vi "BonOMM-SAOMM.Test.vi"() -> ()   [LabVIEW 2011] (continued)
                                n1082 = Bundle("Angle Hor."=w4477, "DEC Tel"=w4476, "Epoch Tel"=w4468) -> (w4475:T29)  [unwired: 1 in]
                                n1083 = flat-sequence {
                                tunnel: w4483 -> [w4491]
                                tunnel: w4478 -> [w4490]
                                tunnel: w4475 -> [w4489]
                                tunnel: w4469 -> [w4488]
                                frame #0 {
                                n1084 = call "Hexapod-Console.vi"("CommCluster"=w4491, "ReferenceCluster"=w4490, "TelescopeCLuster"=w4489, "HexapodCluster"=w4488) -> ()  [unwired: 12 in]
                                }
                                frame #1 {
                                n1085 = local write "HexaSpam"(FALSE ("HexaSpam")) -> ()
                                }
                                }
                                n1086 = while {
                                stop <- w4494 continue-if-true
                                n1087 = Wait (ms)(milliseconds to wait=u32 500) -> ()  [unwired: 1 out]
                                n1088 = local read "HexaSpam"() -> (w4494:bool)
                                n1089 = property on="HexapodRefresh" class="Bool (strict)"("Val(Sgnl)"=TRUE ("Value (Signaling)")) -> ()  [unwired: 2 in, 2 out]
                                }
                                n1090 = Bundle("PrAMS actif"=w4482, "PrAMS-ACK"=w4479, "HexaCons actif"=w4480, "Hexapod-ACK"=w4481) -> (w4478:T30)  [unwired: 1 in]
                              }
                              frame Enabled {
                                n1091 = One Button Dialog(message="Fonction en développement ...\n\nUtilisez plutôt \"déplacement manuel\"") -> ()  [unwired: 1 in, 1 out]
                              }
                            }
                          }
                        }
                      }
                      frame "hex_Paramètres d'asservissement" {
                        # "Ici, on voudra probablement :\n  - Modifier la fréquence du filtre\n  - Modifier le nombre d'image prises en compte\n  - Modifier le coefficient d'aggressivité\n  - Modifier l'affichage de l'historique"
                        n1092 = One Button Dialog(message="Interaction usagé à définir ...") -> ()  [unwired: 1 in, 1 out]
                      }
                      frame "hex_Panneau de offset" {
                        n1093 = flat-sequence {
                          tunnel: [w4504] -> w4498
                          tunnel: w4498 -> [w4511]
                          frame #0 {
                            n1094 = local read "Mode"() -> (w4499:u16)
                            n1095 = case shown="Default" w4499 {
                              frame Default {
                              }
                              frame 0 {
                                n1096 = One Button Dialog(message="Il semble que le système ne soit pas en mode \"collimation\".\n\nPour que les valeurs de offsets demandés prennent effets, il\nest essentiel que le système soit en mode \"collimation\" ou \ntout autre mode utilisant l'hexapode.\n\nPour lancer le mode collimation, lancer d'abord l'exposition\nde la caméra de guidage puis sélectionné \"collimation\".\n\nL'application permettant de charger les offsets d'hexapode\nsera tout de même lancé, mais l'effet ne sera appliqué que\nlors du lancement d'un des modes utilisant l'hexapode.", button name ("OK")="J'ai lu et compris, merci.") -> ()  [unwired: 1 out]
                              }
                            }
                          }
                          frame #1 {
                            n1097 = local write "QueryingHexapod"(TRUE ("Value (Signaling)")) -> ()
                            n1098 = property on="HexapodRefresh" class="Bool (strict)"("Val(Sgnl)"=TRUE ("Value (Signaling)")) -> ()  [unwired: 2 in, 2 out]
                          }
                          frame #2 {
                            n1099 = while {
                              tunnel: [w4505] -> w4504
                              i -> [w4509]
                              stop <- w4508 stop-if-true
                              n1100 = local read "QueryingHexapod"() -> (w4505:bool)
                              n1101 = Not(x=w4505) -> (.not. x?=w4507:bool)
                              n1102 = Wait (ms)(milliseconds to wait=u32 100) -> ()  [unwired: 1 out]
                              n1103 = call "Max-iteration.vi"("i max"=50, "i act"=w4509, "Valeur entrante"=w4507) -> ("break ?"=w4508:bool)
                            }
                          }
                          frame #3 {
                            n1104 = case shown="False" w4511 {
                              frame False {
                                n1105 = control-ref of="Hexapod-ACK"() -> (w4514:refnum<vi>)
                                n1106 = local read "Hexapod VRN"() -> (w4515:refnum<visa-resource-name>)
                                n1107 = control-ref of="Offset X"() -> (w4518:refnum<vi>)
                                n1108 = control-ref of="Offset Y"() -> (w4519:refnum<vi>)
                                n1109 = control-ref of="Offset Z"() -> (w4520:refnum<vi>)
                                n1110 = control-ref of="Offset U"() -> (w4521:refnum<vi>)
                                n1111 = control-ref of="Offset V"() -> (w4522:refnum<vi>)
                                n1112 = local read "MessageType"() -> (w4512:cluster{string[], u32[]})
                                n1113 = control-ref of="HexaCons actif"() -> (w4513:refnum<vi>)
                                n1114 = Bundle("Offset X"=w4518, "Offset Y"=w4519, "Offset Z"=w4520, "Offset U"=w4521, "Offset V"=w4522) -> (w4517:T31)  [unwired: 1 in]
                                n1115 = call "TEST-SAOMM-OffsetGUI.vi"("Hexapod VRN"=w4515, "Active Refnum"=w4513, "PrAMS-ACK"=w4514, "output cluster"=w4517, "MessageType"=w4512) -> ("Error"=w4516:bool)  [unwired: 10 in]
                                n1116 = case shown="True" w4516 {
                                frame False {
                                }
                                frame True {
                                n1117 = One Button Dialog(message="Erreur lors de l'envoi\ndes valeurs de l'offset.") -> ()  [unwired: 1 in, 1 out]
                                }
                                }
                              }
                              frame True {
                                n1118 = One Button Dialog(message="Les valeurs de offsets n'ont pu être lu !?!\nVérifiez la connexion à \"hexapode-console\"") -> ()  [unwired: 1 in, 1 out]
                              }
                            }
                          }
                        }
                      }
                      frame "hex_Déplacement manuel" {
                        n1119 = flat-sequence {
                          tunnel: [w4528] -> w4525
                          tunnel: w4525 -> [w4535]
                          frame #0 {
                            n1120 = local write "QueryingHexapod"(TRUE ("Value (Signaling)")) -> ()
                            n1121 = property on="HexapodRefresh" class="Bool (strict)"("Val(Sgnl)"=TRUE ("Value (Signaling)")) -> ()  [unwired: 2 in, 2 out]
                          }
                          frame #1 {
                            n1122 = while {
                              tunnel: [w4529] -> w4528
                              i -> [w4533]
                              stop <- w4532 stop-if-true
                              n1123 = local read "QueryingHexapod"() -> (w4529:bool)
                              n1124 = Not(x=w4529) -> (.not. x?=w4531:bool)
                              n1125 = Wait (ms)(milliseconds to wait=u32 100) -> ()  [unwired: 1 out]
                              n1126 = call "Max-iteration.vi"("i max"=50, "i act"=w4533, "Valeur entrante"=w4531) -> ("break ?"=w4532:bool)
                            }
                          }
                          frame #2 {
                            n1127 = case shown="False" w4535 {
                              frame False {
                                n1128 = control-ref of="Hexapod-ACK"() -> (w4538:refnum<vi>)
                                n1129 = local read "Hexapod VRN"() -> (w4539:refnum<visa-resource-name>)
                                n1130 = control-ref of="HexX"() -> (w4542:refnum<vi>)
                                n1131 = control-ref of="HexY"() -> (w4543:refnum<vi>)
                                n1132 = control-ref of="HexZ"() -> (w4544:refnum<vi>)
                                n1133 = control-ref of="HexU"() -> (w4545:refnum<vi>)
                                n1134 = control-ref of="HexV"() -> (w4546:refnum<vi>)
                                n1135 = local read "MessageType"() -> (w4536:cluster{string[], u32[]})
                                n1136 = control-ref of="HexaCons actif"() -> (w4537:refnum<vi>)
                                n1137 = Bundle("HexX"=w4542, "HexY"=w4543, "HexZ"=w4544, "HexU"=w4545, "HexV"=w4546) -> (w4541:T28)  [unwired: 1 in]
                                n1138 = call "TEST-SAOMM-PositionGUI.vi"("Hexapod VRN"=w4539, "Active Refnum"=w4537, "PrAMS-ACK"=w4538, "output cluster"=w4541, "MessageType"=w4536) -> ("Error"=w4540:bool)  [unwired: 10 in]
                                n1139 = case shown="True" w4540 {
                                frame False {
                                }
                                frame True {
                                n1140 = One Button Dialog(message="Erreur lors de l'envoi\ndes valeurs de l'offset.") -> ()  [unwired: 1 in, 1 out]
                                }
                                }
                              }
                              frame True {
                                n1141 = One Button Dialog(message="Les valeurs de offsets n'ont pu être lu !?!\nVérifiez la connexion à \"hexapode-console\"") -> ()  [unwired: 1 in, 1 out]
                              }
                            }
                          }
                        }
                      }
                      frame "hex_Remise à zéro" {
                        n1142 = control-ref of="Hexapod-ACK"() -> (w4557:refnum<vi>)
                        n1143 = local read "Hexapod VRN"() -> (w4556:refnum<visa-resource-name>)
                        n1144 = local read "MessageType"() -> (w4553:cluster{string[], u32[]})
                        n1145 = control-ref of="HexaCons actif"() -> (w4558:refnum<vi>)
                        n1146 = local read "HexU"() -> (w4552:dbl)
                        n1147 = local read "HexV"() -> (w4551:dbl)
                        n1148 = local read "Signature"() -> (w4555:u32)
                        n1149 = local read "PrAMS Error"() -> (w4554:errorcluster)
                        n1150 = call "SAOMM-RaZ.vi"("PRAMMS-COMM IN"=w4556, "Active Refnum"=w4558, "PrAMS-ACK"=w4557, "Signature"=w4555, "Error IN"=w4554, "MessageType"=w4553, "Position U"=w4552, "Position V"=w4551) -> ("PRAMMS-COMM OUT"=w4550:refnum<visa-resource-name>, "Error OUT"=w4549:errorcluster)  [unwired: 6 in]
                        n1151 = local write "Hexapod VRN"(w4550) -> ()
                        n1152 = local write "PrAMS Error"(w4549) -> ()
                      }
                    }
                  }
                  frame "main_Caméra de référence" {
                    n1153 = case shown="\"cam_Modifier les paramètres\"" w4560 {
                      selector: w4560 -> [_ _ _ _ w4647 _]
                      tunnel: w4559 -> [_ _ _ _ _ _]
                      frame Default {
                      }
                      frame "cam_Enregistrer la prochaine image" {
                        n1154 = local write "SaveNextImage"(TRUE ("SaveNextImage")) -> ()
                      }
                      frame "cam_Modifier les paramètres" {
                        n1155 = flat-sequence {
                          tunnel: [w4601] -> w4568
                          tunnel: w4568 -> [w4614]
                          tunnel: [w4613] -> w4567
                          tunnel: [w4612] -> w4566
                          tunnel: [w4611] -> w4565
                          tunnel: [w4610] -> w4564
                          tunnel: [w4609] -> w4563
                          tunnel: [w4608] -> w4562
                          frame #0 {
                            n1156 = local write "QueryingPraMS"(TRUE ("Querying")) -> ()
                            n1157 = property on="FalconRefresh" class="Bool (strict)"("Val(Sgnl)"=TRUE ("Value (Signaling)")) -> ()  [unwired: 2 in, 2 out]
                          }
                          frame #1 {
                            n1158 = while {
                              tunnel: [w4603] -> w4601
                              i -> [w4607]
                              stop <- w4606 stop-if-true
                              n1159 = local read "QueryingPraMS"() -> (w4604:bool)
                              n1160 = Not(x=w4604) -> (.not. x?=w4603:bool)
                              n1161 = Wait Until Next ms Multiple(millisecond multiple=u32 50) -> ()  [unwired: 1 out]
                              n1162 = call "Max-iteration.vi"("i max"=100, "i act"=w4607, "Valeur entrante"=w4603) -> ("break ?"=w4606:bool)
                            }
                          }
                          frame #2 {
                            n1163 = case shown="True" w4614 {
                              tunnel: [FALSE ("Apply Changes") w4631] -> w4613
                              tunnel: [u16 0 ("Gain_OUT") w4630] -> w4612
                              tunnel: [u16 0 ("Binning_OUT") w4629] -> w4611
                              tunnel: [0.0 ("FPS_OUT") w4628] -> w4610
                              tunnel: [u16 0 ("Cooling_OUT") w4625] -> w4609
                              tunnel: [0 ("Binning_OUT") w4622] -> w4608
                              frame False {
                                n1164 = One Button Dialog(message="Problème de communication avec Prams") -> ()  [unwired: 1 in, 1 out]
                              }
                              frame True {
                                n1165 = local read "ImageFPS"() -> (w4632:dbl)
                                n1166 = property on="ROIsurface" class="Ring (strict)"() -> ("Strings []"=w4623:string[])  [unwired: 2 in, 2 out]
                                n1167 = local read "FPGA Value"() -> (w4626:u16)
                                n1168 = local read "ROIsurface"() -> (w4624:i32)
                                n1169 = local read "EMGain"() -> (w4627:u16)
                                n1170 = local read "Binning"() -> (w4633:u16)
                                n1171 = call "CameraSettings.vi"("Région d'intérêt"=w4624, "ROIStrings"=w4623, "Gain EM"=w4627, "Refroidissement"=w4626, "Binning"=w4633, "FPS"=w4632) -> ("Apply Changes"=w4631:bool, "Cooling_OUT"=w4625:u16, "Gain_OUT"=w4630:u16, "Binning_OUT"=w4629:u16, "ROISize_OUT"=w4622:i32, "FPS_OUT"=w4628:dbl)  [unwired: 4 in]
                              }
                            }
                          }
                        }
                        n1172 = case shown="True" w4567 {
                          tunnel: w4566 -> [_ w4582]
                          tunnel: w4565 -> [_ w4579]
                          tunnel: w4564 -> [_ w4575]
                          tunnel: w4563 -> [_ w4574]
                          tunnel: w4562 -> [_ w4570]
                          frame False {
                          }
                          frame True {
                            n1173 = flat-sequence {
                              tunnel: [w4588] -> w4583
                              tunnel: w4582 -> [w4588]
                              tunnel: [w4587] -> w4580
                              tunnel: w4579 -> [w4587]
                              tunnel: [w4586] -> w4576
                              tunnel: w4575 -> [w4586]
                              tunnel: w4574 -> [w4585]
                              tunnel: [w4584] -> w4571
                              tunnel: w4570 -> [w4584]
                              tunnel: w4583 -> [w4590]
                              tunnel: [w4592] -> w4581
                              tunnel: w4580 -> [w4592]
                              tunnel: [w4591] -> w4577
                              tunnel: w4576 -> [w4591]
                              tunnel: [w4589] -> w4572
                              tunnel: w4571 -> [w4589]
                              tunnel: w4581 -> [w4594]
                              tunnel: [w4595] -> w4578
                              tunnel: w4577 -> [w4595]
                              tunnel: [w4593] -> w4573
                              tunnel: w4572 -> [w4593]
                              tunnel: w4578 -> [w4597]
                              tunnel: w4573 -> [w4596]
                              tunnel: [w4596] -> w4569
                              tunnel: w4569 -> [w4598]
                              frame #0 {
                                n1174 = property on="FPGA Value" class="Ring (strict)"("Val(Sgnl)"=w4585) -> ()  [unwired: 2 in, 2 out]
                              }
                              frame #1 {
                                n1175 = property on="EMGain" class="DigNum (strict)"("Val(Sgnl)"=w4590) -> ()  [unwired: 2 in, 2 out]
                              }
                              frame #2 {
                                n1176 = property on="Binning" class="Ring (strict)"("Val(Sgnl)"=w4594) -> ()  [unwired: 2 in, 2 out]
                              }
                              frame #3 {
                                n1177 = property on="ImageFPS" class="DigNum (strict)"("Val(Sgnl)"=w4597) -> ()  [unwired: 2 in, 2 out]
                              }
                              frame #4 {
                                n1178 = property on="ROIsurface" class="Ring (strict)"("Val(Sgnl)"=w4598) -> ()  [unwired: 2 in, 2 out]
                              }
                            }
                          }
                        }
                      }
                      frame "cam_Modifier la région d'intérêt" {
                        n1179 = local read "ROIXOffset"() -> (w4644:u16)
                        n1180 = local read "ROIYOffset"() -> (w4643:u16)
                        n1181 = local read "ROIHeight"() -> (w4641:u16)
                        n1182 = local read "ROIWidth"() -> (w4642:u16)
                        n1183 = local read "ImgArray"() -> (w4639:u32[][])
                        n1184 = local read "ROISizes"() -> (w4640:u16[])
                        n1185 = property on="ROIsurface" class="Ring (strict)"() -> ("Strings []"=w4645:string[])  [unwired: 2 in, 2 out]
                        n1186 = call "ROISettings.vi"("ROISizes"=w4640, "SizeEnum"=w4645, "ImgArray"=w4639, "ROIHeight"=w4641, "ROIWidth"=w4642, "ROIYOffset"=w4643, "ROIXOffset"=w4644) -> ("ROIHeightOUT"=w4635:u16, "ROIWidthOUT"=w4636:u16, "ROIYOffsetOUT"=w4637:u16, "ROIXOffsetOUT"=w4638:u16, "SizesOUT"=w4634:i32)
                        n1187 = local write "ROIXOffset"(w4638) -> ()
                        n1188 = local write "ROIYOffset"(w4637) -> ()
                        n1189 = local write "ROIHeight"(w4635) -> ()
                        n1190 = local write "ROIWidth"(w4636) -> ()
                        n1191 = property on="ROIsurface" class="Ring (strict)"("Val(Sgnl)"=w4634) -> ()  [unwired: 2 in, 2 out]
                      }
                      frame "cam_Binning 1x1", "cam_Binning 2x2", "cam_Binning 4x4", "cam_Binning 5x5" {
                        n1192 = case shown="\"cam_Binning 1x1\"" w4647 {
                          tunnel: [u16 1 u16 1 u16 2 u16 4 u16 5] -> w4646
                          frame Default {
                          }
                          frame "cam_Binning 1x1" {
                          }
                          frame "cam_Binning 2x2" {
                          }
                          frame "cam_Binning 4x4" {
                          }
                          frame "cam_Binning 5x5" {
                          }
                        }
                        n1193 = property on="Binning" class="Ring (strict)"("Val(Sgnl)"=w4646) -> ()  [unwired: 2 in, 2 out]
                      }
                      frame "cam_Reconnexion" {
                        n1194 = One Button Dialog(message="Devrait reconnecter Prams ...") -> ()  [unwired: 1 in, 1 out]
                      }
                    }
                  }
                  frame "main_Tables de guidage" {
                    n1195 = case shown="\"tab_Commandes XYZ\"" w4654 {
                      frame Default {
                      }
                      frame "tab_Modifier les vitesses des tables" {
                        # "GUI pour modifier la vitesse des tales ..."
                        n1196 = local read "vitesse lente"() -> (w4660:dbl)
                        n1197 = local read "accelleration"() -> (w4659:dbl)
                        n1198 = local read "vitesse focus"() -> (w4656:dbl)
                        n1199 = local read "vitesse rapide"() -> (w4662:dbl)
                        n1200 = call "Set_table_speed.vi"("Z IN"=w4656, "Accel IN"=w4659, "Fast IN"=w4662, "slow IN"=w4660) -> ("Z OUT"=w4655:dbl, "Accel OUT"=w4657:dbl, "Fast OUT"=w4661:dbl, "slow OUT"=w4658:dbl)  [unwired: 4 in]
                        n1201 = local write "vitesse rapide"(w4661) -> ()
                        n1202 = local write "accelleration"(w4657) -> ()
                        n1203 = local write "vitesse focus"(w4655) -> ()
                        n1204 = local write "vitesse lente"(w4658) -> ()
                      }
                      frame "tab_Positions prédéfinies" {
                        n1205 = local read "Rangement X"() -> (w4672:dbl)
                        n1206 = local read "Rangement Y"() -> (w4673:dbl)
                        n1207 = local read "Rangement Z"() -> (w4671:dbl)
                        n1208 = local read "Calibration X"() -> (w4682:dbl)
                        n1209 = local read "Calibration Y"() -> (w4681:dbl)
                        n1210 = local read "Reference X"() -> (w4679:dbl)
                        n1211 = local read "Reference Y"() -> (w4678:dbl)
                        n1212 = local read "CentreTel X"() -> (w4676:dbl)
                        n1213 = local read "CentreTel Y"() -> (w4675:dbl)
                        n1214 = local read "Position X"() -> (w4670:dbl)
                        n1215 = local read "Position Y"() -> (w4669:dbl)
                        n1216 = Bundle("CentreTel X"=w4676, "CentreTel Y"=w4675) -> (w4674:cluster{"CentreTel X":dbl, "CentreTel Y":dbl})  [unwired: 1 in]
                        n1217 = Bundle("Reference X"=w4679, "Reference Y"=w4678) -> (w4677:cluster{"Reference X":dbl, "Reference Y":dbl})  [unwired: 1 in]
                        n1218 = Bundle("Calibration X"=w4682, "Calibration Y"=w4681) -> (w4680:T32)  [unwired: 1 in]
                        n1219 = Bundle("Rangement X"=w4672, "Rangement Y"=w4673, "Rangement Z"=w4671) -> (w4666:T33)  [unwired: 1 in]
                        n1220 = call "Set_predefined_table_positions.vi"("Calibration IN"=w4680, "Position Y"=w4669, "Position X"=w4670, "Reference IN"=w4677, "Centre IN"=w4674, "Park IN"=w4666) -> ("Calibration OUT"=w4667:T34, "Reference OUT"=w4663:cluster{"Reference Y":dbl, "Reference X":dbl}, "Centre OUT"=w4664:cluster{"Centre Y":dbl, "Centre X":dbl}, "Accept?"=w4668:bool, "Park OUT"=w4665:T35)  [unwired: 5 in]
                        n1221 = case shown="True" w4668 {
                          tunnel: w4667 -> [_ w4695]
                          tunnel: w4665 -> [_ w4692]
                          tunnel: w4664 -> [_ w4688]
                          tunnel: w4663 -> [_ w4685]
                          frame False {
                          }
                          frame True {
                            n1222 = Unbundle(w4695) -> ("Calibration Y"=w4694:dbl, "Calibration X"=w4693:dbl)
                            n1223 = Unbundle(w4688) -> ("Centre Y"=w4687:dbl, "Centre X"=w4686:dbl)
                            n1224 = Unbundle(w4685) -> ("Reference Y"=w4684:dbl, "Reference X"=w4683:dbl)
                            n1225 = Unbundle(w4692) -> ("Range Y"=w4691:dbl, "Range X"=w4690:dbl, "Range Z"=w4689:dbl)
                            n1226 = local write "Rangement X"(w4691) -> ()
                            n1227 = local write "Rangement Y"(w4690) -> ()
                            n1228 = local write "Rangement Z"(w4689) -> ()
                            n1229 = local write "Calibration X"(w4694) -> ()
                            n1230 = local write "Calibration Y"(w4693) -> ()
                            n1231 = local write "Reference X"(w4684) -> ()
                            n1232 = local write "Reference Y"(w4683) -> ()
                            n1233 = local write "CentreTel X"(w4687) -> ()
                            n1234 = local write "CentreTel Y"(w4686) -> ()
                          }
                        }
                      }
                      frame "tab_Commandes XYZ" {
                        n1235 = local read "MovingZ"() -> (w4698:bool)
                        n1236 = local read "MovingXY"() -> (w4697:bool)
                        n1237 = Or(x=w4698, y=w4697) -> (x .or. y?=w4696:bool)
                        n1238 = case shown="False" w4696 {
                          frame False {
                            n1239 = control-ref of="Table VRN"() -> (w4702:refnum<vi>)
                            n1240 = control-ref of="Table Error"() -> (w4701:refnum<vi>)
                            n1241 = control-ref of="Table actif"() -> (w4700:refnum<vi>)
                            n1242 = control-ref of="Cible X"() -> (w4705:refnum<vi>)
                            n1243 = control-ref of="Cible Y"() -> (w4706:refnum<vi>)
                            n1244 = control-ref of="Cible Z"() -> (w4704:refnum<vi>)
                            n1245 = local read "Position X"() -> (w4709:dbl)
                            n1246 = local read "Position Y"() -> (w4708:dbl)
                            n1247 = local read "Position Z"() -> (w4707:dbl)
                            n1248 = Bundle("Cible X"=w4705, "Cible Y"=w4706, "Cible Z"=w4704) -> (w4703:T36)  [unwired: 1 in]
                            n1249 = Bundle("Table VRN"=w4702, "Table Error"=w4701, "Table actif"=w4700) -> (w4699:T37)  [unwired: 1 in]
                            n1250 = call "CommandesXYZ.vi"("Structure-Communications"=w4699, "Structure-Cibles"=w4703, "Position X"=w4709, "Position Y"=w4708, "Position Z"=w4707) -> ()  [unwired: 11 in]
                          }
                          frame True {
                            n1251 = One Button Dialog(message="Les tables de translation semblent déjà être\nen mouvement, assurez-vous qu'elles sont arrêtées\navant de lancer le mode \"XYZ\".") -> ()  [unwired: 1 in, 1 out]
                          }
                        }
                      }
                      frame "tab_Modifier les paramètres" {
                        # "ClickJOG est en minute d'arc ..."
                        n1252 = local read "ClickJOG"() -> (w4714:dbl)
                        n1253 = expression code="x*60.0"(w4714) -> (w4713:dbl)
                        n1254 = call "Set-Jog-Params.vi"("clic IN"=w4713) -> ("clic OUT"=w4712:dbl)  [unwired: 14 in]
                        n1255 = expression code="x/60.0"(w4712) -> (w4711:dbl)
                        n1256 = local write "ClickJOG"(w4711) -> ()
                      }
                      frame "Reconnexion" {
                      }
                    }
                  }
                  frame "main_Roue à filtres" {
                    n1257 = case shown="\"raf_Reconnexion\"" w4715 {
                      selector: w4715 -> [w4721 _ _]
                      frame Default {
                        w4719 = "@@"
                        # "hmm, à compléter ...\n\n  - Cocher le filtre en place\n  - Commencer par rafraichir\n  - Si déconnecté, ne pas permettre un déplacement de la roue ..."
                        n1258 = Search/Split String(string=w4721, search string/char (-)=w4719) -> (match + rest of string=w4720:string)  [unwired: 1 in, 2 out]
                        n1259 = String Length(string=w4719) -> (length=w4718:i32)
                        n1260 = String Subset(string=w4720, offset (0)=w4718) -> (substring=w4717:string)  [unwired: 1 in]
                        n1261 = Decimal String To Number(string=w4717) -> (number=w4716:i32)  [unwired: 2 in, 1 out]
                        n1262 = Greater Or Equal To 0?(x=w4716) -> (x >= 0?=w4722:bool)
                        n1263 = case shown="True" w4722 {
                          tunnel: w4716 -> [_ w4734]
                          frame False {
                          }
                          frame True {
                            n1264 = Replace Array Subset(array=bool[] [FALSE, FALSE, FALSE, FALSE, FALSE, FALSE], new element=TRUE ("new element/subarray"), index=w4734) -> (w4728:bool[])
                            n1265 = property on="ChoixFiltre" class="Clust (strict)"() -> ("Value"=w4731:T12)  [unwired: 2 in, 2 out]
                            n1266 = Index Array(array=w4728) -> (element #1=w4729:bool, element #2=w4727:bool, element #3=w4726:bool, element #4=w4725:bool, element #5=w4724:bool, element #6=w4723:bool)  [unwired: 6 in]
                            n1267 = Bundle(cluster=w4731, "filtre #1"=w4729, "filtre #2"=w4727, "filtre #3"=w4726, "filtre #4"=w4725, "filtre #5"=w4724, "filtre #6"=w4723) -> (w4730:T12)
                            n1268 = property on="ChoixFiltre" class="Clust (strict)"("Val(Sgnl)"=w4730) -> ()  [unwired: 2 in, 2 out]
                          }
                        }
                      }
                      frame "raf_Modifier la liste des filtres" {
                        n1269 = flat-sequence {
                          frame #0 {
                            n1270 = local write "HautDroit"(T11."Périphérique" ("HautDroit")) -> ()
                          }
                          frame #1 {
                            n1271 = property on="change_filtre_liste" class="Bool (strict)"("Val(Sgnl)"=TRUE) -> ()  [unwired: 2 in, 2 out]
                          }
                        }
                      }
                      frame "raf_Reconnexion" {
                        n1272 = flat-sequence {
                          frame #0 {
                            w4738 = u16 0 items=["Roue à Filtres (BonOMM)", "Roue à Filtres (PANO-II)", "Foyer ST-133", "Lampes d'étalonnage", "Options des périphériques"] ("Périphérique")
                            n1273 = local write "HautDroit"(T11."Périphérique" ("HautDroit")) -> ()
                            n1274 = local write "Périphérique"(w4738) -> ()
                          }
                          frame #1 {
                            n1275 = property on="reconnect" class="Bool (strict)"("Val(Sgnl)"=TRUE ("Value (Signaling)")) -> ()  [unwired: 2 in, 2 out]
                          }
                        }
                      }
                    }
                  }
                }
              }
              event Key Down {
                n1276 = event-data() -> ("Char"=w4740:i16, "ScanCode"=w4741:i16)  [unwired: 1 in, 7 out]
                n1277 = case shown="0" w4740 {
                  tunnel: w4741 -> [_ w4742 _ _ _ _ _ _]
                  frame Default {
                    # "Do nothing ..."
                  }
                  frame 0 {
                    n1278 = case shown="72, 75, 77, 80" w4742 {
                      selector: w4742 -> [_ w4744]
                      frame Default {
                      }
                      frame 72, 75, 77, 80 {
                        # "Les 4 flèches ..."
                        # "Passer dans une astrométrie ?"
                        n1279 = local read "Servo"() -> (w4743:bool)
                        n1280 = case shown="False" w4743 {
                          tunnel: w4744 -> [w4758 _]
                          frame False {
                            # "Va marcher seulement 99.9% du temps, les SETs doivent être directement\nici si on veut éviter que ProcessedFalconImage ne puisse venir modifier\nles paramètres avant l'envoi."
                            n1281 = property on="ImgArray" class="IntGraph (strict)"("Active Cursor"=u32 0) -> (error out=w4755:errorcluster)  [unwired: 2 in, 1 out]
                            n1282 = property on="ImgArray" class="IntGraph (strict)"(error in=w4755) -> ("Cursor.Cursor X"=w4757:dbl, "Cursor.Cursor Y"=w4756:dbl)  [unwired: 1 in, 2 out]
                            n1283 = case shown="Default" w4758 {
                              tunnel: w4757 -> [w4763 w4764 w4768 w4772 w4775]
                              tunnel: w4756 -> [w4762 w4766 w4769 w4771 w4773]
                              tunnel: [w4763 w4764 w4767 w4772 w4774] -> w4753
                              tunnel: [w4762 w4765 w4769 w4770 w4773] -> w4752
                              frame Default {
                              }
                              frame 72 {
                                # "\"Up\""
                                n1284 = Increment(x=w4766) -> (x+1=w4765:dbl)
                              }
                              frame 77 {
                                # "\"Right\""
                                n1285 = Increment(x=w4768) -> (x+1=w4767:dbl)
                              }
                              frame 80 {
                                # "\"Down\""
                                n1286 = Decrement(x=w4771) -> (x-1=w4770:dbl)
                              }
                              frame 75 {
                                # "\"Left\""
                                n1287 = Decrement(x=w4775) -> (x-1=w4774:dbl)
                              }
                            }
                            n1288 = local read "ROIWidth"() -> (w4751:u16)
                            n1289 = local read "ROIHeight"() -> (w4750:u16)
                            n1290 = control-ref of="ImgArray"() -> (w4745:refnum<vi>)
                            n1291 = call "SAOMM-Cursor2ROI.vi"("ImgRef"=w4745, "CursorX"=w4753, "CursorY"=w4752, "ROIWidth"=w4751, "ROIHeight"=w4750) -> ("XÉtoile"=w4746:dbl, "YÉtoile"=w4747:dbl, "ROIXOffset"=w4749:u16, "ROIYOffset"=w4748:u16)  [unwired: 7 in]
                            n1292 = local write "XReference"(w4746) -> ()
                            n1293 = local write "YReference"(w4747) -> ()
                            n1294 = flat-sequence {
                              tunnel: w4749 -> [w4760]
                              tunnel: w4748 -> [w4759]
                              frame #0 {
                                n1295 = local write "ROIXOffset"(w4760) -> ()
                                n1296 = local write "ROIYOffset"(w4759) -> ()
                              }
                              frame #1 {
                                n1297 = property on="UpdateROI" class="Bool (strict)"("Val(Sgnl)"=TRUE ("Value (Signaling)")) -> ()  [unwired: 2 in, 2 out]
                              }
                            }
                          }
                          frame True {
                            n1298 = One Button Dialog(message="Vous ne pouvez pas modifier la ROI pendant l'asservissement") -> ()  [unwired: 1 in, 1 out]
                          }
                        }
                      }
                    }
                  }
                  frame 9 {
                    # "tab"
                    n1299 = property on="Offset OK" class="Bool (strict)"() -> ("Key Focus"=w4777:bool)  [unwired: 2 in, 2 out]
                    n1300 = property on="N.O. A.D." class="Str"() -> ("Key Focus"=w4781:bool)  [unwired: 2 in, 2 out]
                    n1301 = property on="N.O. Déc." class="Str"() -> ("Key Focus"=w4782:bool)  [unwired: 2 in, 2 out]
                    n1302 = property on="NO epoch" class="DigNum (strict)"() -> ("Key Focus"=w4783:bool)  [unwired: 2 in, 2 out]
                    n1303 = property on="ModCoor" class="Bool (strict)"() -> ("Key Focus"=w4784:bool)  [unwired: 2 in, 2 out]
                    n1304 = property on="Offset RA" class="DigNum (strict)"() -> ("Key Focus"=w4779:bool)  [unwired: 2 in, 2 out]
                    n1305 = property on="Offset DEC" class="DigNum (strict)"() -> ("Key Focus"=w4778:bool)  [unwired: 2 in, 2 out]
                    n1306 = Compound Arithmetic op=OR(w4781, w4782, w4783, w4784, w4779, w4778, w4777) -> (w4780:bool)
                    n1307 = case shown="False" w4780 {
                      frame False {
                        n1308 = flat-sequence {
                          frame #0 {
                            n1309 = property on="N.O. A.D." class="Str"("Key Focus"=TRUE) -> ()  [unwired: 2 in, 2 out]
                          }
                          frame #1 {
                            n1310 = property on="NO RA clic-sim" class="Bool (strict)"("Val(Sgnl)"=TRUE ("Value (Signaling)")) -> ()  [unwired: 2 in, 2 out]
                          }
                        }
                      }
                      frame True {
                      }
                    }
                  }
                  frame 32 {
                    # "Space bar"
                    n1311 = property on="Obslib" class="Tbl (strict)"() -> ("Key Focus"=w4787:bool)  [unwired: 2 in, 2 out]
                    n1312 = case shown="False" w4787 {
                      frame False {
                        n1313 = property on="Offset RA" class="DigNum (strict)"("Key Focus"=TRUE) -> ()  [unwired: 2 in, 2 out]
                      }
                      frame True {
                      }
                    }
                  }
                  frame 101 {
                    # "'e' pour Est"
                    n1314 = local read "Offset RA"() -> (w4790:dbl)
                    n1315 = Absolute Value(x=w4790) -> (abs(x)=w4789:dbl)
                    n1316 = property on="Offset RA" class="DigNum (strict)"("Val(Sgnl)"=w4789) -> ()  [unwired: 2 in, 2 out]
                  }
                  frame 110 {
                    # "'n' pour Nord"
                    n1317 = local read "Offset DEC"() -> (w4792:dbl)
                    n1318 = Absolute Value(x=w4792) -> (abs(x)=w4791:dbl)
                    n1319 = property on="Offset DEC" class="DigNum (strict)"("Val(Sgnl)"=w4791) -> ()  [unwired: 2 in, 2 out]
                  }
                  frame 111, 119 {
                    # "'o' ou 'w' pour Ouest"
                    n1320 = local read "Offset RA"() -> (w4795:dbl)
                    n1321 = Absolute Value(x=w4795) -> (abs(x)=w4794:dbl)
                    n1322 = Negate(x=w4794) -> (-x=w4793:dbl)
                    n1323 = property on="Offset RA" class="DigNum (strict)"("Val(Sgnl)"=w4793) -> ()  [unwired: 2 in, 2 out]
                  }
                  frame 115 {
                    # "'s' pour Sud"
                    n1324 = local read "Offset DEC"() -> (w4798:dbl)
                    n1325 = Absolute Value(x=w4798) -> (abs(x)=w4797:dbl)
                    n1326 = Negate(x=w4797) -> (-x=w4796:dbl)
                    n1327 = property on="Offset DEC" class="DigNum (strict)"("Val(Sgnl)"=w4796) -> ()  [unwired: 2 in, 2 out]
                  }
                }
              }
              event Mouse Move {
                n1328 = event-data() -> ()  [unwired: 1 in, 4 out]
                n1329 = disable-structure shown="Enabled" {
                  frame Disabled {
                    n1330 = while {
                      stop <- w4802 continue-if-true
                      w4803 = -1 ("x")
                      n1331 = property on="Picture" class="Pict"() -> ("Mouse"=w4806:T38)  [unwired: 2 in, 2 out]
                      n1332 = Unbundle By Name(w4806) -> ("Mouse Position.X"=w4801:i32, "Mouse Position.Y"=w4800:i32, "Mouse Modifiers.Button Down"=w4799:bool)
                      n1333 = case shown="True" w4799 {
                        frame False {
                        }
                        frame True {
                          n1334 = control-ref of="ImgArray"() -> (w4807:refnum<vi>)
                          n1335 = local write "Naxis1"(i16 640 ("Nx")) -> ()
                          n1336 = local write "Naxis2"(i16 480 ("Ny")) -> ()
                          n1337 = local write item#-1(i16 0 ("Xs")) -> ()
                          n1338 = local write item#-1(i16 0 ("Ys")) -> ()
                          n1339 = stacked-sequence {
                            seq-local: [w4813 _] -> [_ w4873]
                            seq-local: [w4812 _] -> [_ w4872]
                            tunnel: w4807 -> [w4814 _]
                            frame #0 {
                              n1340 = while {
                                tunnel: w4814 -> [w4817]
                                tunnel: [w4816] -> w4813
                                tunnel: [w4815] -> w4812
                                i -> [w4819]
                                stop <- w4818 continue-if-true
                                n1341 = property on="Picture" class="Pict"() -> ("Mouse"=w4821:T38)  [unwired: 2 in, 2 out]
                                n1342 = Equal To 0?(x=w4819) -> (x = 0?=w4820:bool)
                                n1343 = Unbundle By Name(w4821) -> ("Mouse Position.X"=w4816:i32, "Mouse Position.Y"=w4815:i32, "Mouse Modifiers.Button Down"=w4818:bool)
                                n1344 = case shown="False" w4820 {
                                tunnel: w4816 -> [w4823 w4861]
                                tunnel: w4815 -> [w4822 w4842]
                                tunnel: w4817 -> [w4834 w4860]
                                frame False {
                                # "Correspond à la grandeur du picture pas de la caméra de guidage ..."
                                n1345 = local read item#-1() -> (w4839)
                                n1346 = local read item#-1() -> (w4840)
                                n1347 = Bundle(w4840, w4839, "X"=w4823, "Y"=w4822) -> (w4841:cluster{void, void, "X":i32, "Y":i32})  [unwired: 1 in]
                                n1348 = property class="IntGraph (strict)"(reference=w4834, "Active Cursor"=u32 0) -> ("Y Scale.Range:Maximum"=w4825:dbl, "Y Scale.Range:Minimum"=w4824:dbl, "X Scale.Range:Maximum"=w4836:dbl, "X Scale.Range:Minimum"=w4835:dbl)  [unwired: 1 in, 2 out]
                                n1349 = call "BoxCrossPict.vi"("rect"=w4841) -> ("Pict Out"=→"Picture":picture)  [unwired: 1 in, 2 out]
                                n1350 = control-ref of="Picture"() -> (w4832:refnum<vi>)
                                n1351 = property class="Pict"(reference=w4832) -> ("Draw Area Size"=w4833:T39)  [unwired: 1 in, 2 out]
                                n1352 = Unbundle(w4833) -> ("Width"=w4829:u32, "Height"=w4828:u32)
                                n1353 = Subtract(x=w4828, y=u32 6) -> (x-y=w4830:u32)
                                n1354 = Subtract(x=w4829, y=u32 6) -> (x-y=w4831:u32)
                                n1355 = call "Pict_to_Graph.vi"("Xo"=w4823, "Width"=w4831, "Yo"=w4822, "Heigth"=w4830, "X Scale.Range:Minimum"=w4835, "X Scale.Range:Maximum"=w4836, "Y Scale.Range:Minimum"=w4824, "Y Scale.Range:Maximum"=w4825) -> ()  [unwired: 2 in, 2 out]
                                }
                                frame True {
                                n1356 = property class="IntGraph (strict)"(reference=w4860, "Active Cursor"=u32 0) -> (reference out=w4852:refnum<vi>, "Y Scale.Range:Maximum"=w4856:dbl, "Y Scale.Range:Minimum"=w4855:dbl, "X Scale.Range:Maximum"=w4854:dbl, "X Scale.Range:Minimum"=w4853:dbl)  [unwired: 1 in, 1 out]
                                n1357 = control-ref of="Picture"() -> (w4849:refnum<vi>)
                                n1358 = property class="Pict"(reference=w4849) -> ("Draw Area Size"=w4850:T39)  [unwired: 1 in, 2 out]
                                n1359 = Unbundle(w4850) -> ("Width"=w4848:u32, "Height"=w4847:u32)
                                n1360 = Subtract(x=w4847, y=u32 6) -> (x-y=w4843:u32)
                                n1361 = Subtract(x=w4848, y=u32 6) -> (x-y=w4844:u32)
                                n1362 = call "Pict_to_Graph.vi"("Xo"=w4861, "Width"=w4844, "Yo"=w4842, "Heigth"=w4843, "X Scale.Range:Minimum"=w4853, "X Scale.Range:Maximum"=w4854, "Y Scale.Range:Minimum"=w4855, "Y Scale.Range:Maximum"=w4856) -> ("CursorY"=w4858:dbl, "CursorX"=w4859:dbl)  [unwired: 2 in]
                                n1363 = property class="IntGraph (strict)"(reference=w4852, "Active Cursor"=u32 0, "Cursor.Cursor Position:Cursor X"=w4859, "Cursor.Cursor Position:Cursor Y"=w4858) -> ()  [unwired: 1 in, 2 out]
                                }
                                }
                              }
                            }
                            frame #1 {
                              n1364 = local read item#-1() -> (w4877)
                              n1365 = local read item#-1() -> (w4874)
                              n1366 = Max & Min(x=w4877, y=w4873) -> (min(x,y)=w4871:i32)  [unwired: 1 out]
                              n1367 = Max & Min(x=w4872, y=w4874) -> (max(x,y)=w4862:i32)  [unwired: 1 out]
                              n1368 = control-ref of="ImgArray"() -> (w4863:refnum<vi>)
                              n1369 = Subtract(x=w4877, y=w4873) -> (x-y=w4875:i32)
                              n1370 = Subtract(x=w4872, y=w4874) -> (x-y=w4876:i32)
                              n1371 = control-ref of="Picture"() -> (w4864:refnum<vi>)
                              n1372 = Absolute Value(x=w4875) -> (abs(x)=w4870:i32)
                              n1373 = Absolute Value(x=w4876) -> (abs(x)=w4869:i32)
                              n1374 = call "PICT_to_CAM.vi"("Pict Refnum"=w4864, "IntGraph Refnum"=w4863, "Ny"=w4869, "Yo"=w4862, "Nx"=w4870, "Xo"=w4871) -> ("Ny CAM"=→"Naxis2":i16, "Nx CAM"=→"Naxis1":i16, "Yo CAM"=w4867:i16, "Xo CAM"=w4868:i16)
                            }
                          }
                        }
                      }
                      n1375 = Not Equal?(x=w4801, y=w4803) -> (x != y?=w4804:bool)
                      n1376 = Not Equal?(x=w4803, y=w4800) -> (x != y?=w4805:bool)
                      n1377 = And(x=w4804, y=w4805) -> (x .and. y?=w4802:bool)
                    }
                  }
                  frame Enabled {
                  }
                }
              }
              event "TableXYPos": Cursor Grab {
                n1378 = event-data() -> ("CursIdx"=w4879:i32)  [unwired: 1 in, 7 out]
                n1379 = stacked-sequence {
                  tunnel: w4879 -> [w4880 _ _]
                  frame #0 {
                    n1380 = property on="TableXYPos" class="XYGraph (strict)"("Active Cursor"=w4880) -> ()  [unwired: 2 in, 2 out]
                    n1381 = case shown="1" w4880 {
                      tunnel: [TRUE FALSE] -> w4882
                      tunnel: [FALSE TRUE] -> w4881
                      frame 1 {
                      }
                      frame 0, Default {
                      }
                    }
                    n1382 = local write "act_cible"(w4881) -> ()
                    n1383 = local write "act_sonde"(w4882) -> ()
                  }
                  frame #1 {
                    n1384 = local read "ImgData"() -> (w4887:sgl[][])
                    n1385 = while {
                      tunnel: w4887 -> [w4890]
                      stop <- w4888 stop-if-true
                      n1386 = event shown="[0] Timeout" {
                        selector: _ -> [_ _]
                        dyn-events: _ -> [_ _]
                        timeout: 100 -> [_ _]
                        tunnel: w4890 -> [_ _]
                        tunnel: [FALSE TRUE] -> w4888
                        event Timeout {
                          w4891 = u16 1 items=["Region d'intérêt", "Prévisualisation"] ("ImageUsage")
                          n1387 = event-data() -> ()  [unwired: 1 in, 2 out]
                          n1388 = property on="TableXYPos" class="XYGraph (strict)"("Active Cursor"=u32 0) -> (error out=w4895:errorcluster)  [unwired: 2 in, 1 out]
                          n1389 = local read "FieldAstrom"() -> (w4897:T4)
                          n1390 = property on="TableXYPos" class="XYGraph (strict)"(error in=w4895) -> ("Cursor.Cursor X"=w4903:dbl, "Cursor.Cursor Y"=w4902:dbl)  [unwired: 1 in, 2 out]
                          n1391 = call "xy2ad.vi"("Y (px)"=w4902, "X (px)"=w4903, "Astrometry"=w4897) -> ("DEC (°)"=w4899:dbl, "RA (°)"=w4900:dbl, "DEC (HH:MM:SS)"=w4901:dbl, "RA (HH:MM:SS.S)"=w4898:dbl)  [unwired: 5 in]
                          n1392 = local read "ImgAstrom"() -> (w4911:T4)
                          n1393 = local write "RA Cible"(w4898) -> ()
                          n1394 = local write "Dec Cible"(w4901) -> ()
                          n1395 = local read "ImgData"() -> (w4904:sgl[][])
                          n1396 = call "ad2xy.vi"("DEC"=w4899, "RA"=w4900, "Astrometry"=w4911) -> ("Y"=w4910:dbl, "X"=w4909:dbl)  [unwired: 6 in, 1 out]
                          n1397 = To Long Integer(number=w4909) -> (32bit integer=w4906:i32)
                          n1398 = To Long Integer(number=w4910) -> (32bit integer=w4905:i32)
                          n1399 = call "subimage.vi"("Ysz/2"=100 ("Xsz/2"), "Xsz/2"=100, "Yc"=w4905, "Xc"=w4906, "ImgData"=w4904) -> ("SubImg"=w4893:sgl[][])  [unwired: 6 in]
                          n1400 = Array Max & Min(array=w4893) -> (max value=w4892:sgl)  [unwired: 3 out]
                          n1401 = call "Draw_crosshair.vi"("Image IN"=w4893, "White Value"=w4892) -> ("Image OUT"=→"subimg":sgl[][])  [unwired: 13 in]
                          n1402 = local write "ImageUsage"(w4891) -> ()
                        }
                        event "TableXYPos": Cursor Release {
                          n1403 = event-data() -> ()  [unwired: 1 in, 8 out]
                        }
                      }
                    }
                  }
                  frame #2 {
                    n1404 = local write "CursorGrab"(FALSE ("CursorGrab")) -> ()
                  }
                }
                "CursorGrab" <- TRUE ("CursorGrab")
              }
              event "RA Cible", "Dec Cible", "RA Sonde", "Dec Sonde", "act_cible", "act_sonde": Mouse Down {
                n1405 = event-data() -> ("CtlRef"=w4918:refnum<vi>)  [unwired: 1 in, 6 out]
                n1406 = property class="Ctl"(reference=w4918) -> ("Label.Text"=w4917:string)  [unwired: 1 in, 2 out]
                n1407 = case shown="\"Dec Cible\", \"RA Cible\", \"act_cible\", Default" w4917 {
                  tunnel: [TRUE FALSE] -> w4915
                  tunnel: [FALSE TRUE] -> w4916
                  frame "Dec Sonde", "RA Sonde", "act_sonde" {
                  }
                  frame "Dec Cible", "RA Cible", "act_cible", Default {
                  }
                }
                "act_sonde" <- w4915
                "act_cible" <- w4916
              }
              event "N.O. A.D.", "N.O. Déc.", "NO epoch": Value Change {
                # "Peut-être qu'ici on"
                n1408 = event-data() -> ()  [unwired: 1 in, 6 out]
                n1409 = local read "N.O. Déc."() -> (w4936:string)
                n1410 = local read "N.O. A.D."() -> (w4937:string)
                n1411 = call "format_coords_str(new).vi"("DEC str"=w4936, "RA str"=w4937) -> ("%s DEC"=w4934:string, "%s RA"=w4935:string)  [unwired: 1 in]
                n1412 = local read "NO epoch"() -> (w4933:dbl)
                n1413 = call "time-str-to-time-dbl-RA.vi"("Chaîne"=w4935) -> ("TCS_coords"=w4926:dbl)
                n1414 = call "time-str-to-time-dbl-DEC.vi"("Chaîne"=w4934) -> ("TCS_coords"=w4924:dbl)
                n1415 = local read "LST"() -> (w4932:dbl)
                n1416 = expression code="x*3600"(w4926) -> (w4925:dbl)
                n1417 = expression code="x*3600"(w4924) -> (w4923:dbl)
                n1418 = call "Object_properties.vi"("Target RA"=w4925, "Target DEC"=w4923, "Target Epoch"=w4933, "Sideral Time"=w4932) -> ("NO RA"=w4931:string, "NO DEC"=w4930:string, "NO Epoch"=w4928:dbl, "NO HA"=w4927:dbl, "NO AM"=w4929:dbl)  [unwired: 7 in]
                n1419 = local write "NO AM"(w4929) -> ()
                n1420 = local write "NO HA"(w4927) -> ()
                n1421 = local write "NO epoch"(w4928) -> ()
                n1422 = local write "N.O. Déc."(w4930) -> ()
                n1423 = local write "N.O. A.D."(w4931) -> ()
              }
              event "Flat": Value Change {
                n1424 = event-data() -> ("NewVal"=w4941:bool)  [unwired: 1 in, 4 out]
                n1425 = Select(t="Ouverture" ("Indicateur d'état"), s=w4941, f="Fermeture" ("Indicateur d'état")) -> (s? t:f=w4945:string)
                n1426 = local read "Calib VRN"() -> (w4949:refnum<visa-resource-name>)
                n1427 = Concatenate Strings(w4945, " de la lampe de flat" ("Indicateur d'état")) -> (w4948:string)
                n1428 = control-ref of="TERMINAL"() -> (w4942:refnum<vi>)
                n1429 = control-ref of="Indicateur d'état"() -> (w4943:refnum<vi>)
                n1430 = Build Array("Arc", "Néon", w4941) -> (w4950:bool[])
                n1431 = call "Controle_des_lampe.vi"("VISA resource name"=w4949, "Status In"=w4950) -> ("Status Out"=w4940:bool[])  [unwired: 2 out]
                n1432 = local write "Status lamp"(w4940) -> ()
                n1433 = call "TERMINAL.vi"("Indicateur Refnum"=w4943, "Terminal Refnum"=w4942, "Indicateur d'état"=w4948) -> ()
                n1434 = Index Array(array=w4940, index=0 ("Index")) -> (element=→"ArcOn":bool)
                n1435 = Index Array(array=w4940, index=1 ("Index")) -> (element=→"NeonOn":bool)
                n1436 = Index Array(array=w4940, index=2 ("Index")) -> (element=→"FlatOn":bool)
                n1437 = Boolean Array To Number(Boolean array=w4940) -> (number=w4939:u32)
                n1438 = Greater Than 0?(x=w4939) -> (x > 0?=w4938:bool)
                n1439 = property on="lampOn?" class="Bool (strict)"("Blinking"=w4938, "Visible"=w4938) -> ()  [unwired: 2 in, 2 out]
              }
              event "Néon": Value Change {
                n1440 = event-data() -> ("NewVal"=w4962:bool)  [unwired: 1 in, 4 out]
                n1441 = local read "Arc"() -> (w4979:bool)
                n1442 = Select(t="Ouverture" ("Indicateur d'état"), s=w4962, f="Fermeture" ("Indicateur d'état")) -> (s? t:f=w4966:string)
                n1443 = Build Array(w4979, w4962, "Flat") -> (w4972:bool[])
                n1444 = local read "Calib VRN"() -> (w4970:refnum<visa-resource-name>)
                n1445 = Concatenate Strings(w4966, " de la lampe de Néon" ("Indicateur d'état")) -> (w4963:string)
                n1446 = call "Controle_des_lampe.vi"("VISA resource name"=w4970, "Status In"=w4972) -> ("Status Out"=w4959:bool[])  [unwired: 2 out]
                n1447 = local write "Status lamp"(w4959) -> ()
                n1448 = control-ref of="TERMINAL"() -> (w4969:refnum<vi>)
                n1449 = control-ref of="Indicateur d'état"() -> (w4968:refnum<vi>)
                n1450 = call "TERMINAL.vi"("Indicateur Refnum"=w4968, "Terminal Refnum"=w4969, "Indicateur d'état"=w4963) -> ()
                n1451 = Boolean Array To Number(Boolean array=w4959) -> (number=w4960:u32)
                n1452 = Index Array(array=w4959, index=0 ("Index")) -> (element=w4976:bool)
                n1453 = Index Array(array=w4959, index=1 ("Index")) -> (element=w4977:bool)
                n1454 = Index Array(array=w4959, index=2 ("Index")) -> (element=w4978:bool)
                n1455 = Greater Than 0?(x=w4960) -> (x > 0?=w4961:bool)
                n1456 = local write "NeonOn"(w4977) -> ()
                n1457 = local write "ArcOn"(w4976) -> ()
                n1458 = local write "FlatOn"(w4978) -> ()
                n1459 = property on="lampOn?" class="Bool (strict)"("Blinking"=w4961, "Visible"=w4961) -> ()  [unwired: 2 in, 2 out]
              }
              event "Arc": Value Change {
                n1460 = event-data() -> ("NewVal"=w4983:bool)  [unwired: 1 in, 4 out]
                n1461 = local read "Néon"() -> (w5000:bool)
                n1462 = local read "Flat"() -> (w4992:bool)
                n1463 = Select(t="Ouverture" ("Indicateur d'état"), s=w4983, f="Fermeture" ("Indicateur d'état")) -> (s? t:f=w4987:string)
                n1464 = Build Array(w4983, w5000, w4992) -> (w4993:bool[])
                n1465 = local read "Calib VRN"() -> (w4991:refnum<visa-resource-name>)
                n1466 = call "Controle_des_lampe.vi"("VISA resource name"=w4991, "Status In"=w4993) -> ("Status Out"=w4980:bool[])  [unwired: 2 out]
                n1467 = local write "Status lamp"(w4980) -> ()
                n1468 = Concatenate Strings(w4987, " de la lampe à arc" ("Indicateur d'état")) -> (w4984:string)
                n1469 = control-ref of="TERMINAL"() -> (w4990:refnum<vi>)
                n1470 = control-ref of="Indicateur d'état"() -> (w4989:refnum<vi>)
                n1471 = Index Array(array=w4980, index=0 ("Index")) -> (element=w4997:bool)
                n1472 = Index Array(array=w4980, index=1 ("Index")) -> (element=w4998:bool)
                n1473 = Index Array(array=w4980, index=2 ("Index")) -> (element=w4999:bool)
                n1474 = Boolean Array To Number(Boolean array=w4980) -> (number=w4982:u32)
                n1475 = call "TERMINAL.vi"("Indicateur Refnum"=w4989, "Terminal Refnum"=w4990, "Indicateur d'état"=w4984) -> ()
                n1476 = Greater Than 0?(x=w4982) -> (x > 0?=w4981:bool)
                n1477 = local write "NeonOn"(w4998) -> ()
                n1478 = local write "ArcOn"(w4997) -> ()
                n1479 = local write "FlatOn"(w4999) -> ()
                n1480 = property on="lampOn?" class="Bool (strict)"("Blinking"=w4981, "Visible"=w4981) -> ()  [unwired: 2 in, 2 out]
              }
              event "ModCoor": Value Change {
                n1481 = event-data() -> ("NewVal"=w5002:bool)  [unwired: 1 in, 4 out]
                n1482 = case shown="True" w5002 {
                  tunnel: [FALSE w5005] -> w5001
                  frame False {
                  }
                  frame True {
                    # "Système acquisition ou\ntechnicien est prioritaire"
                    # "Epoque=0=>courante du TCS"
                    n1483 = call "time-str-to-time-dbl-DEC.vi"("Chaîne"="N.O. Déc.") -> ("TCS_coords"=w5014:dbl)
                    n1484 = call "time-str-to-time-dbl-RA.vi"("Chaîne"="N.O. A.D.") -> ("TCS_coords"=w5013:dbl)
                    n1485 = control-ref of="TERMINAL"() -> (w5021:refnum<vi>)
                    n1486 = control-ref of="Indicateur d'état"() -> (w5022:refnum<vi>)
                    n1487 = control-ref of="TCS actif"() -> (w5006:refnum<vi>)
                    n1488 = Concatenate Strings("Chargement des coordonnées : ", "N.O. A.D.", ", ", "N.O. Déc.") -> (w5016:string)
                    n1489 = local read "TCS VRN"() -> (w5011:refnum<visa-resource-name>)
                    n1490 = Build Array(w5013, w5014, "NO epoch") -> (w5012:dbl[])
                    n1491 = call "TERMINAL.vi"("Indicateur Refnum"=w5022, "Terminal Refnum"=w5021, "Indicateur d'état"=w5016) -> ()
                    n1492 = call "EXCOM-CMD.vi"("VRN IN"=w5011, "Bool Refnum"=w5006, "Commande #"=6, "Args"=w5012) -> ("VRN OUT"=w5007:refnum<visa-resource-name>, "OK Done"=w5009:bool, "Error OUT"=w5008:errorcluster)  [unwired: 9 in]
                    n1493 = local write "ModCoor"(FALSE) -> ()
                    n1494 = local write "TCS Error"(w5008) -> ()
                    n1495 = local write "TCS VRN"(w5007) -> ()
                    n1496 = case shown="True" w5009 {
                      tunnel: [FALSE w5027] -> w5005
                      frame False {
                        n1497 = One Button Dialog(message="ATTENTION!!\nProblème d'écriture\ndes nouvelles coordonnées.\nVérifiez TCS.", button name ("OK")="OK" ("nom du bouton (\"OK\")")) -> ()  [unwired: 1 out]
                      }
                      frame True {
                        w5027 = TRUE
                        n1498 = local read "STATL"() -> (w5028:bool[])
                        n1499 = Index Array(array=w5028, index=2 ("Index")) -> ()  [unwired: 1 out]
